vi "Window Memory write from DMA - Target.vi"   [LabVIEW 2014]
uses:
  <vilib>/rvi/Emulation/niFpgaGetClockAttributes.vi
  <vilib>/rvi/Emulation/niFpgaSctlEmulationGetInTimedLoop.vi
  <vilib>/rvi/Emulation/niFpgaEmulationReportErrorSimple.vi
  <vilib>/rvi/interface/RandomDataEmulation/niFpgaRandomDataHandleErrors.vi
  <vilib>/rvi/Memory/Memory_Emulation/nirvimemoryFastEmulation.vi
  <vilib>/rvi/Memory/Memory_Emulation/nirvimemoryEmulation.vi
  <vilib>/rvi/Emulation/niFpgaEmulationIsFPGAContextNoSignature.vi
  <vilib>/rvi/DataTransferAndStorage/Container/Common/niFpgaContainerGetUniqueNameForEmu.vi
  <vilib>/rvi/Emulation/niFpgaProcessEmulError.vi
  <vilib>/rvi/errors/nirviReportUnexpectedCaseInternalError (U32).vi
  <vilib>/rvi/Emulation/niFpgaCriticalErrorInLSC.vi
  <vilib>/rvi/DataTransferAndStorage/Container/XNode/niFpgaContainer.xnode
  <vilib>/rvi/interface/RandomDataEmulation/nirviRandomDataFpgaReadWriteTemplate.vi
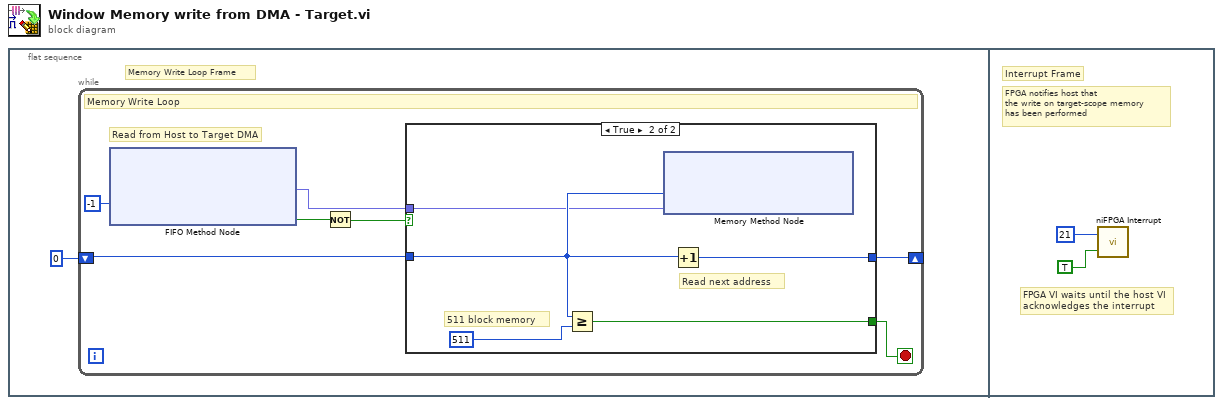
[diagram p0: block diagram]
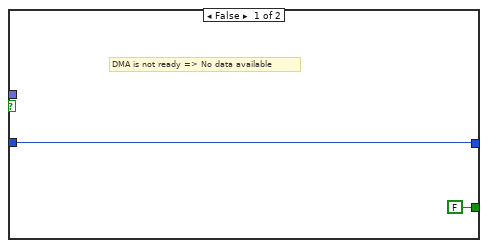
[diagram p2: hidden frame]
diagram:
  n1 = flat-sequence {
    frame #0 {
      # "Memory Write Loop Frame"
      n2 = while {
        shift-right: [w6] -> _
        shift-left: u32 0 -> [w7]
        stop <- w8 stop-if-true
        # "Read from Host to Target DMA"
        # "Memory Write Loop"
        n3 = xnode ("FIFO Method Node")("Timeout"=-1) -> ("Element"=w2:fxp<+,8,1>, "Timed Out?"=w4:bool)  [unwired: 1 in, 1 out]
        n4 = Not(x=w4) -> (.not. x?=w3:bool)
        n5 = case shown="True" w3 {
          tunnel: [FALSE w14] -> w8
          tunnel: w7 -> [w9 w13]
          tunnel: [w9 w12] -> w6
          tunnel: w2 -> [_ w11]
          frame False {
            # "DMA is not ready => No data available"
          }
          frame True {
            # "Read next address"
            # "511 block memory"
            n6 = Greater Or Equal?(x=w13, y=u32 511) -> (x >= y?=w14:bool)
            n7 = xnode ("Memory Method Node")("Address"=w13, "Data"=w11) -> ()  [unwired: 1 in, 1 out]
            n8 = Increment(x=w13) -> (x+1=w12:u32)
          }
        }
      }
    }
    frame #1 {
      # "FPGA VI waits until the host VI \nacknowledges the interrupt"
      # "FPGA notifies host that\nthe write on target-scope memory\nhas been performed"
      # "Interrupt Frame"
      n9 = call <vilib>:"niFPGA Interrupt.vi"("Wait Until Cleared (F)"=TRUE, "IRQ Number (0)"=u8 21) -> ()  [unwired: 1 in]
    }
  }
